vi "Read Depth Data.vi"(8 "error in (no error)":errorcluster, 11 "Depth Data Message in":refnum<class "Depth Data Message.lvclass">) -> (0 "error out":errorcluster, 2 "Depth Data":T1, 3 "Depth Data Message out":refnum<class "Depth Data Message.lvclass">)   [LabVIEW 2015, in "RDS Child Messages.lvlib" / "Depth Data Message.lvclass"]
uses:
  Depth Data Message.lvclass
  Depth Data.ctl
  Depth Data Message.lvclass/Depth Data Message.ctl
  RDS Child Messages.lvlib
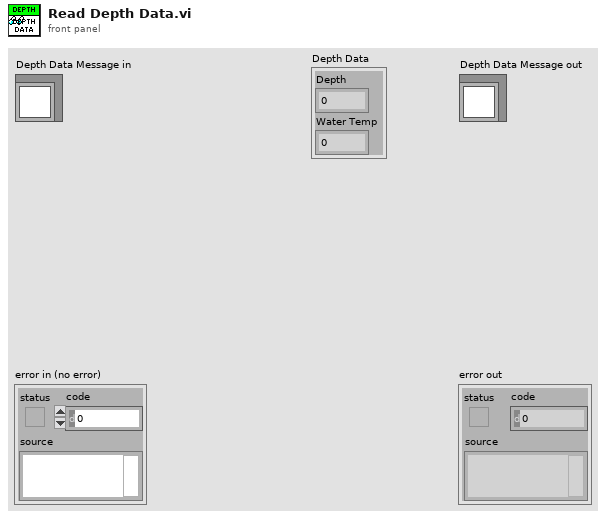
[diagram p1: front panel]
types:
  T1 = typedef "RDS Child Messages.lvlib/Depth Data.ctl" = cluster{"Depth":sgl, "Water Temp":i8}
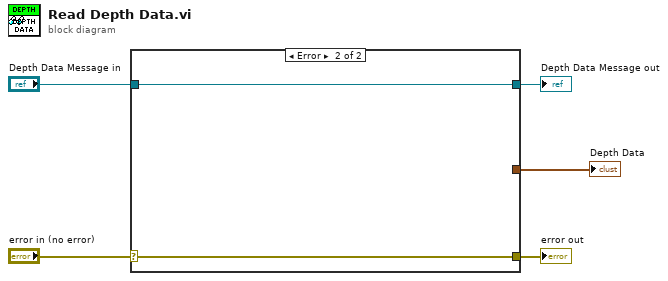
[diagram p0: block diagram]
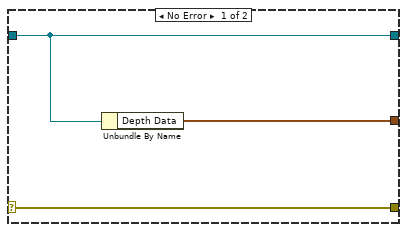
[diagram p2: hidden frame]
diagram:
  n1 = case shown="Error" "error in (no error)" {
    selector: "error in (no error)" -> [w8 w9]
    tunnel: [w8 w9] -> w4
    tunnel: [w7 w10] -> w2
    tunnel: "Depth Data Message in" -> [w7 w10]
    tunnel: [w6 _] -> w1
    frame No Error {
      n2 = Unbundle By Name(w7) -> ("Depth Data"=w6:T1)
    }
    frame Error {
    }
  }
  "error out" <- w4
  "Depth Data Message out" <- w2
  "Depth Data" <- w1
